vi "SDG60UploadArbWaveform.vi"(4 "WFM Source":u16(ring) items=["Single file", "Split files", "Array"], 5 "WFM (Column) Number":i32, 6 "Array WFM":i16[](array[numeric])=[1000, 2000, 3000, 4000, 5000, 6000, 7000, 8000], 7 "WFM Length (20E6)":i32=20000000, 8 "error in (no error)":errorcluster, 9 "Timeout (40000 ms)":u32=40000, 10 "Waveform Numer ARB1":u32=1, 11 "VISA resource name":refnum<visa-resource-name>="USB0::0xF4EC::0x1101::SDG6XEBC5R0119::INSTR") -> (0 "error out":errorcluster, 1 "Total time":dbl format="%#_15g", 3 "VISA resource name out":refnum<visa-resource-name>)   [LabVIEW 2018]
doc: "Creates and saves an arbitrary (user-defined) waveform in non-volatile memory, then selects it for output."
uses:
  <vilib>/Utility/file.llb/Read From Spreadsheet File (I64).vi
panel:
  out "Check String":string
  out "WFM to arr time":dbl format="%#_15g"
  out "Arr to str time":dbl format="%#_15g"
  out "Upload time":dbl format="%#_15g"
  out "Attempts (0: First)":i32
  in  "WFM Path":path=path "C:/Data/_SoftDevelopment/SDG6000/WFMTst20E6PtsInt.txt"
  # "The input range for ARB data is: -32767..+32767 (must be integers)\n\nC1 hardcoded within vi as needs to have a channel assigned to be uploaded. \nCan then be selected for either channel.\n\nUpon overwrite of name with new WFM, still needs to be selected\notherwise will still use old WFM with that name. If WFM has been selected, and then gets deleted off \nC drive, will still output WFM on that channel\n\nTesting uploads of large WFMS.\n8M: All ok, can have 2 separate WFMs on 2 channels and upload more\n16M: Can have 2 separate WFMs on 2 channels, storage space limits 3rd upload\n          of 16M points, but can upload 8M and switch fine between them all.\n20M: Can have 20M on both channels, but then no storage space to upload third\n\nVi will write the file with a small (16B bin file on device) file (overwriting any WFM \n           previously with that name),  then write the WFM selected with the one chosen to \n           upload.  This means you don't need to clear space off the device, as long as the \n           name of the WFM is already on the device. If a new name is chosen, then will have to manually delete the old WFM, \n           or use SDG60DeleteAllWaveforms vi, if need to free up space.\n\nIf too large a waveform is uploaded (over 20M), generator will crash requiring manual power\ncycle\n\nIf storage full, will beep on generator and say storage full, but not give any error through \nlabview. Waveform won't ovewrite others when uploading if storage full.\n\nSingle pixel test, (oscilloscope limited to 200MHz) , for 20M points. the single pixel did go to\n +32767, Pk-Pk on scope was 3.36V when should be 4.0 Vpp. The burst width (FWHM) was \n3.962 ns. RMS was 1.99 V. 3.2ns FWHM on 2GHz infiinium scope (no longer limited by scope)"
  # "Max: 20E6 (decimal)"
  # "TODO:  cab adopt\nreadback (see AWG5200)"
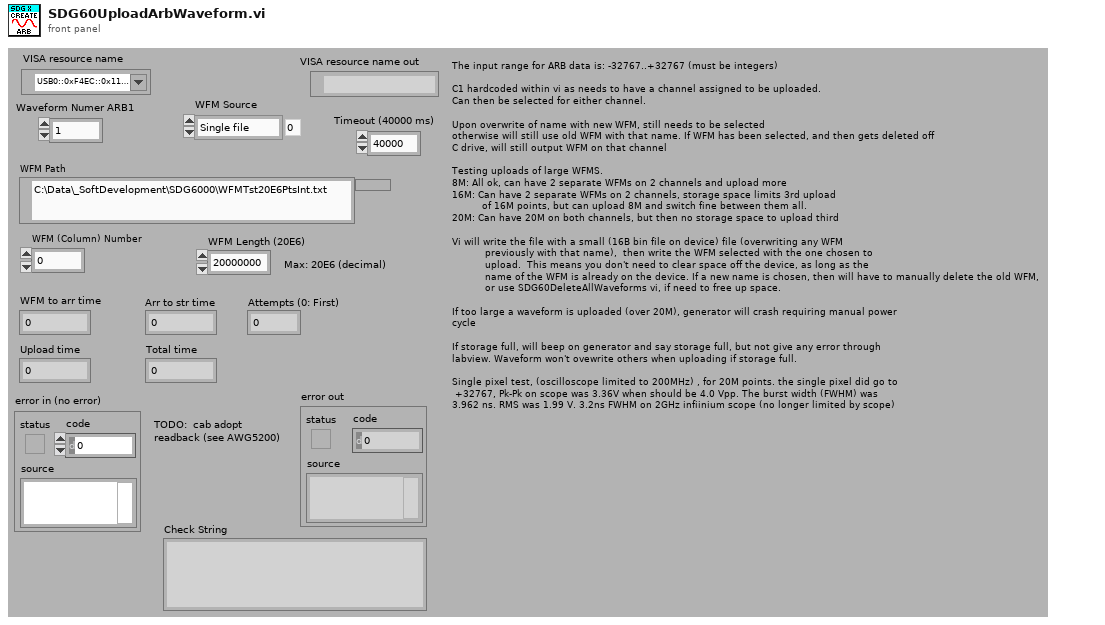
[diagram p1: front panel]
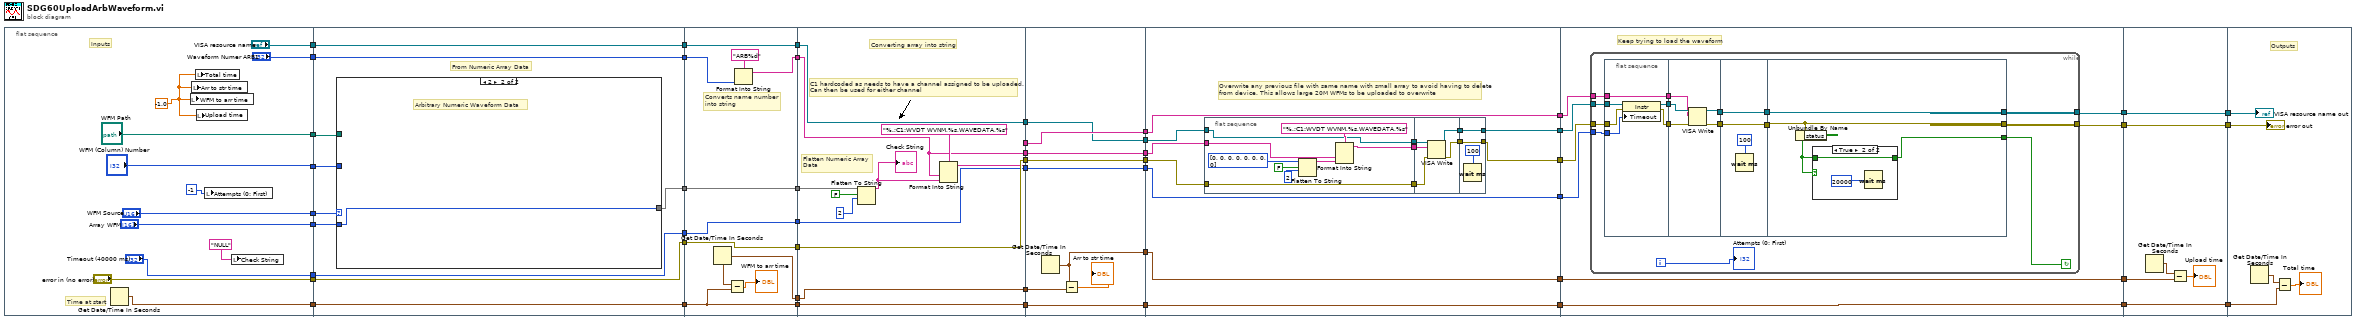
[diagram p0: block diagram]
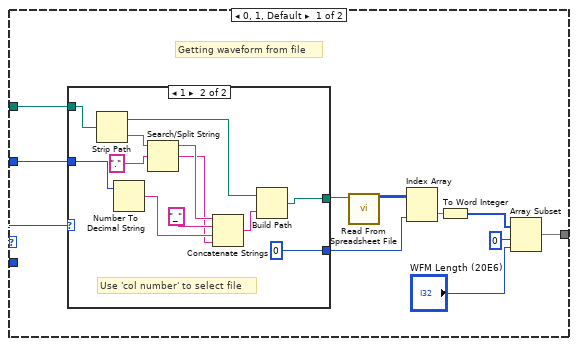
[diagram p2: hidden frame]
diagram:
  n1 = flat-sequence {
    tunnel: ["WFM Source"] -> w9
    tunnel: ["Array WFM"] -> w8
    tunnel: ["WFM Path"] -> w7
    tunnel: ["WFM (Column) Number"] -> w6
    tunnel: ["VISA resource name"] -> w5
    tunnel: ["error in (no error)"] -> w3
    tunnel: ["Timeout (40000 ms)"] -> w2
    tunnel: [w54] -> w1
    tunnel: ["Waveform Numer ARB1"] -> w4
    tunnel: w9 -> [w71]
    tunnel: w8 -> [w70]
    tunnel: [w69] -> w49
    tunnel: w7 -> [w68]
    tunnel: w6 -> [w67]
    tunnel: [w66] -> w47
    tunnel: w5 -> [w66]
    tunnel: [w65] -> w45
    tunnel: w4 -> [w65]
    tunnel: [w64] -> w43
    tunnel: w3 -> [w64]
    tunnel: [w63] -> w41
    tunnel: w2 -> [w63]
    tunnel: [w62] -> w39
    tunnel: w1 -> [w62]
    tunnel: w49 -> [w107]
    tunnel: [w107] -> w48
    tunnel: w47 -> [w106]
    tunnel: [w106] -> w46
    tunnel: w45 -> [w98]
    tunnel: [w99] -> w44
    tunnel: w43 -> [w102]
    tunnel: [w102] -> w42
    tunnel: w41 -> [w103]
    tunnel: [w103] -> w40
    tunnel: w39 -> [w104]
    tunnel: [w104] -> w38
    tunnel: [w101] -> w24
    tunnel: w48 -> [w111]
    tunnel: [w113] -> w37
    tunnel: [w118] -> w36
    tunnel: [w117] -> w35
    tunnel: [w116] -> w34
    tunnel: w46 -> [w118]
    tunnel: w44 -> [w108]
    tunnel: w42 -> [w117]
    tunnel: w40 -> [w116]
    tunnel: w38 -> [w115]
    tunnel: [w115] -> w33
    tunnel: [w114] -> w25
    tunnel: w24 -> [w114]
    tunnel: [w108] -> w10
    tunnel: w37 -> [w128]
    tunnel: [w128] -> w23
    tunnel: w36 -> [w127]
    tunnel: [w127] -> w21
    tunnel: w35 -> [w126]
    tunnel: [w126] -> w19
    tunnel: w34 -> [w125]
    tunnel: [w125] -> w17
    tunnel: w33 -> [w121]
    tunnel: [w121] -> w15
    tunnel: [w123] -> w13
    tunnel: w25 -> [w122]
    tunnel: [w120] -> w11
    tunnel: w10 -> [w120]
    tunnel: w23 -> [w142]
    tunnel: [w142] -> w22
    tunnel: w21 -> [w130]
    tunnel: [w129] -> w20
    tunnel: w19 -> [w134]
    tunnel: [w133] -> w18
    tunnel: w17 -> [w141]
    tunnel: [w141] -> w16
    tunnel: w15 -> [w140]
    tunnel: [w140] -> w14
    tunnel: w13 -> [w139]
    tunnel: [w139] -> w12
    tunnel: w11 -> [w138]
    tunnel: [w163] -> w32
    tunnel: [w162] -> w30
    tunnel: w22 -> [w167]
    tunnel: w20 -> [w166]
    tunnel: w18 -> [w165]
    tunnel: w16 -> [w164]
    tunnel: w14 -> [w161]
    tunnel: [w161] -> w28
    tunnel: w12 -> [w160]
    tunnel: [w160] -> w26
    tunnel: w32 -> [w209]
    tunnel: [w209] -> w31
    tunnel: w30 -> [w208]
    tunnel: [w208] -> w29
    tunnel: w28 -> [w206]
    tunnel: [w206] -> w27
    tunnel: w26 -> [w205]
    tunnel: w31 -> [w214]
    tunnel: w29 -> [w213]
    tunnel: w27 -> [w210]
    frame #0 {
      w53 = -1.0
      # "Inputs"
      # "Time at start"
      n2 = Get Date/Time In Seconds() -> (seconds since 1Jan1904=w54:timestamp)
      n3 = local write "WFM to arr time"(w53) -> ()
      n4 = local write "Arr to str time"(w53) -> ()
      n5 = local write "Total time"(w53) -> ()
      n6 = local write "Upload time"(w53) -> ()
      n7 = local write "Attempts (0: First)"(-1) -> ()
      n8 = local write "Check String"("NULL") -> ()
    }
    frame #1 {
      # "From Numeric Array Data"
      n9 = case shown="2" w71 {
        selector: w71 -> [w80 _]
        tunnel: [w75 w97] -> w69
        tunnel: w70 -> [_ w97]
        tunnel: w68 -> [w74 _]
        tunnel: w67 -> [w73 _]
        frame 0, 1, Default {
          # "Getting waveform from file"
          n10 = case shown="1" w80 {
            tunnel: w74 -> [w84 w96]
            tunnel: w73 -> [w83 w93]
            tunnel: [w84 w86] -> w78
            tunnel: [w83 0 ("x")] -> w77
            frame 0, Default {
              # "File contains multiple wfms"
            }
            frame 1 {
              # "Use 'col number' to select file"
              n11 = Strip Path(path=w96) -> (stripped path=w88:path, name=w94:string)
              n12 = Number To Decimal String(number=w93) -> (decimal integer string=w90:string)  [unwired: 1 in]
              n13 = Search/Split String(string=w94, search string/char (-)=".") -> (substring before match=w92:string, match + rest of string=w89:string)  [unwired: 1 in, 1 out]
              n14 = Concatenate Strings(w92, "_", w90, w89) -> (w87:string)
              n15 = Build Path(base path=w88, name or relative path=w87) -> (appended path=w86:path)
            }
          }
          n16 = call-poly <vilib>:"Read From Spreadsheet File.vi"("file path (dialog if empty)"=w78) -> ("all rows"=w79:i64[][])  [unwired: 6 in, 4 out]
          n17 = Index Array(array=w79, index (col)=w77) -> (element=w76:i64[])  [unwired: 1 in]
          n18 = To Word Integer(number=w76) -> (16bit integer=w82:i16[])
          n19 = Array Subset(array=w82, index=0 ("x"), length="WFM Length (20E6)") -> (w75:i16[])
        }
        frame 2 {
          # "Arbitrary Numeric Waveform Data"
        }
      }
    }
    frame #2 {
      # "Converts name number \ninto string"
      n20 = Get Date/Time In Seconds() -> (seconds since 1Jan1904=w101:timestamp)
      n21 = Subtract(x=w101, y=w104) -> (x-y=→"WFM to arr time":dbl)
      n22 = Format Into String(format string="ARB%d", w98) -> (resulting string=w99:string)  [unwired: 2 in, 1 out]
    }
    frame #3 {
      # "Converting array into string"
      # "C1 hardcoded as needs to have a channel assigned to be uploaded. \nCan then be used for either channel"
      # "Flatten Numeric Array \nData"
      n23 = Flatten To String(anything=w111, prepend array or string size? (T)=FALSE, byte order (0:big-endian, network order)=2) -> (data string=w109:string)  [unwired: 1 in, 2 out]
      "Check String" <- w109
      n24 = Format Into String(format string="%.;C1:WVDT WVNM,%s,WAVEDATA,%s", w108, w109) -> (resulting string=w113:string)  [unwired: 2 in, 1 out]
    }
    frame #4 {
      n25 = Get Date/Time In Seconds() -> (seconds since 1Jan1904=w123:timestamp)
      n26 = Subtract(x=w123, y=w122) -> (x-y=→"Arr to str time":dbl)
    }
    frame #5 {
      # "Overwrite any previous file with same name with small array to avoid having to delete\nfrom device. This allows large 20M WFMs to be uploaded to overwrite"
      n27 = flat-sequence {
        tunnel: w138 -> [w150]
        tunnel: [w145] -> w137
        tunnel: w134 -> [w144]
        tunnel: [w144] -> w136
        tunnel: w130 -> [w143]
        tunnel: [w143] -> w132
        tunnel: w137 -> [w156]
        tunnel: w136 -> [w155]
        tunnel: [w154] -> w135
        tunnel: w132 -> [w153]
        tunnel: [w152] -> w131
        tunnel: [w158] -> w133
        tunnel: w135 -> [w158]
        tunnel: [w157] -> w129
        tunnel: w131 -> [w157]
        frame #0 {
          n28 = Flatten To String(anything=i16[] [0, 0, 0, 0, 0, 0, 0, 0] ("Array WFM DUMMY"), prepend array or string size? (T)=FALSE, byte order (0:big-endian, network order)=2) -> (data string=w147:string)  [unwired: 1 in, 2 out]
          n29 = Format Into String(format string="%.;C1:WVDT WVNM,%s,WAVEDATA,%s", w150, w147) -> (resulting string=w145:string)  [unwired: 2 in, 1 out]
        }
        frame #1 {
          n30 = VISA Write(VISA resource name=w153, write buffer=w156, error in (no error)=w155) -> (VISA resource name out=w152:refnum<visa-resource-name>, error out=w154:errorcluster)  [unwired: 1 out]
        }
        frame #2 {
          n31 = Wait (ms)(milliseconds to wait=100 ("x")) -> ()  [unwired: 1 out]
        }
      }
    }
    frame #6 {
      # "Keep trying to load the waveform"
      n32 = while {
        tunnel: w167 -> [w182]
        tunnel: w166 -> [w181]
        tunnel: w165 -> [w180]
        tunnel: [w179] -> w163
        tunnel: [w178] -> w162
        tunnel: w164 -> [w168]
        i -> [w174]
        stop <- w177 continue-if-true
        n33 = flat-sequence {
          tunnel: w182 -> [w188]
          tunnel: w180 -> [w185]
          tunnel: w181 -> [w187]
          tunnel: [w186] -> w171
          tunnel: [w184] -> w170
          tunnel: [w188] -> w169
          tunnel: w168 -> [w183]
          tunnel: [w189] -> w176
          tunnel: [w190] -> w175
          tunnel: w171 -> [w192]
          tunnel: w170 -> [w193]
          tunnel: w169 -> [w191]
          tunnel: w176 -> [w194]
          tunnel: w175 -> [w195]
          tunnel: [w195] -> w173
          tunnel: [w194] -> w172
          tunnel: [w198] -> w178
          tunnel: [w197] -> w179
          tunnel: [w199] -> w177
          tunnel: w173 -> [w198]
          tunnel: w172 -> [w197]
          frame #0 {
            n34 = property class="Instr"(reference=w187, error in=w185, "Timeout"=w183) -> (reference out=w186:refnum<visa-resource-name>, error out=w184:errorcluster)
          }
          frame #1 {
            n35 = VISA Write(VISA resource name=w192, write buffer=w191, error in (no error)=w193) -> (VISA resource name out=w190:refnum<visa-resource-name>, error out=w189:errorcluster)  [unwired: 1 out]
          }
          frame #2 {
            n36 = Wait (ms)(milliseconds to wait=100 ("x")) -> ()  [unwired: 1 out]
          }
          frame #3 {
            n37 = Unbundle By Name(w197) -> ("status"=w200:bool)
            n38 = case shown="True" w200 {
              tunnel: w200 -> [w201 w202]
              tunnel: [w201 w202] -> w199
              frame False {
              }
              frame True {
                n39 = Wait (ms)(milliseconds to wait=20000 ("x")) -> ()  [unwired: 1 out]
              }
            }
          }
        }
        "Attempts (0: First)" <- w174
      }
    }
    frame #7 {
      n40 = Get Date/Time In Seconds() -> (seconds since 1Jan1904=w207:timestamp)
      n41 = Subtract(x=w207, y=w205) -> (x-y=→"Upload time":dbl)
    }
    frame #8 {
      # "Outputs"
      n42 = Get Date/Time In Seconds() -> (seconds since 1Jan1904=w212:timestamp)
      n43 = Subtract(x=w212, y=w210) -> (x-y=→"Total time":dbl)
      "VISA resource name out" <- w213
      "error out" <- w214
    }
  }
